vi "AssignItemContent.vi"(8 "error in (no error)":errorcluster, 9 "Category hierarchy[]":string[](array[string]), 10 "Folder hierarchy[]":string[](array[string]), 11 "CLabVIEWItemLLB in":refnum<class "CLabVIEWItemLLB.lvclass">) -> (0 "error out":errorcluster, 3 "CLabVIEWItemLLB out":refnum<class "CLabVIEWItemLLB.lvclass">)   [LabVIEW 2020, in "LabVIEWContainers.lvlib" / "CLabVIEWItemLLB.lvclass"]
uses:
  CLabVIEWItemLLB.lvclass
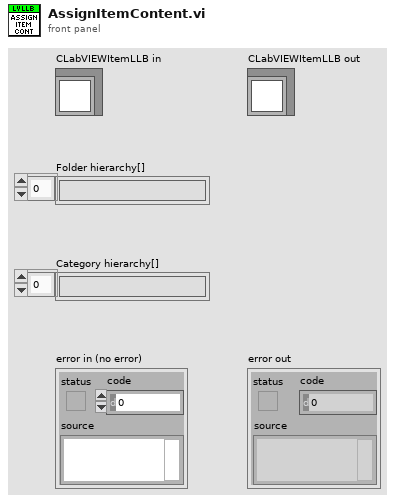
[diagram p1: front panel]
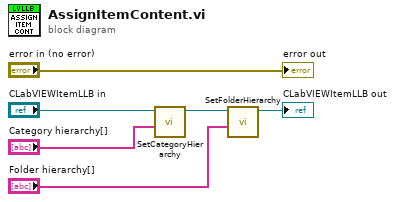
[diagram p0: block diagram]
diagram:
  n1 = call-dynamic "SetCategoryHierarchy.vi"("Category hierarchy[]"="Category hierarchy[]", "CLabVIEWItem in"="CLabVIEWItemLLB in") -> ("CLabVIEWItem out"=w5:refnum<class "CLabVIEWItemLLB.lvclass">)  [unwired: 8 in, 1 out]
  n2 = call-dynamic "SetFolderHierarchy.vi"("Folder hierarchy[]"="Folder hierarchy[]", "CLabVIEWItem in"=w5) -> ("CLabVIEWItem out"=→"CLabVIEWItemLLB out":refnum<class "CLabVIEWItemLLB.lvclass">)  [unwired: 8 in, 1 out]
  "error out" <- "error in (no error)"
